vi "test code emballage_PAGO.vi"() -> ()   [LabVIEW 2011]
uses:
  <vilib>/Instr/_visa.llb/VISA Configure Serial Port (Instr).vi
panel:
  in  "Param RS232 2":T1={"VISA resource name"="COM4", "baud rate"=9600, "data bits"=8, "parity"=0, "stop bits"=10, "flow control"=0, "delay before read (ms)"=500} {"data bits" min=5 max=8 step=1; "parity" items=["Aucune", "Impaire", "Paire", "Marque", "Espace"]; "stop bits" items=["1.0"=10, "1.5"=15, "2.0"=20]; "flow control" items=["Aucune"=0, "XON/XOFF"=1, "RTS/CTS"=2, "DTR/DSR"=4]}
  in  "chaine ecrite":string
  out "chaine lue":string
  in  "Param RS232":T1={"VISA resource name"="COM4", "baud rate"=9600, "data bits"=8, "parity"=0, "stop bits"=10, "flow control"=0, "delay before read (ms)"=500} {"data bits" min=5 max=8 step=1; "parity" items=["Aucune", "Impaire", "Paire", "Marque", "Espace"]; "stop bits" items=["1.0"=10, "1.5"=15, "2.0"=20]; "flow control" items=["Aucune"=0, "XON/XOFF"=1, "RTS/CTS"=2, "DTR/DSR"=4]}
  # "ENTETE LOGO FAS MEDIC"
  # "ZB\nUS\nq592\nD7\nN\nR166,48\nI8,12,001\nGW275,824,30,55,ÿÿÿÿÿÿÿÿÿÿÿÿÿÿÿÿÿÿÿÿÿÿÿÿÿÿÿÿùÿÿÿÿÿÿÿÿÿÿÿÿÿÿÿÿÿÿÿÿÿÿÿÿÿÿÿÿÿàÿÿÿÿÿÿÿÿÿÿÿÿÿÿÿÿÿÿÿÿÿÿÿÿÿÿÿÿÿÿÿÿÿÿÿÿÿÿÿÿÿÿÿÿÿÿÿÿÿÿÿÿÿÿÿÿÿþÿÿÿÿÿÿÿÿÿÿÿÿÿÿÿÿÿÿÿÿÿÿÿÿÿÿÿø?ÿÿÿÿÿÿÿÿÿÿÿÿÿÿÿÿÿÿÿÿÿÿÿÿÿÿÿð?ÿÿÿÿÿÿÿÿÿÿÿÿÿÿÿÿÿÿÿÿÿÿÿÿÿÿÿð?ÿÿÿÿÿÿÿÿÿÿÿÿÿÿÿÿÿÿÿÿÿÿÿÿÿÿÿðÿÿÿÿÿÿÿÿÿÿÿÿÿÿÿÿÿÿÿÿÿÿÿÿÿÿÿàÿÿÿÿÿÿÿÿÿÿÿÿÿÿÿÿÿÿÿÿÿÿÿÿÿÿÿÀÿÿÿÿÿÿÿÿÿÿÿÿÿÿÿÿÿÿÿÿÿÿÿÿÿÿÿÀ?ÿàÿÿþÿàÿÿÿÿÿÿÀÿÿðÿÿÿÿÿÿÿÀ?ÿ?Ïxÿ?þóþþÀÿ?ü?þÏaàþþóø>?øüÇÏGü|Çþóð??ðüÿãÏOþxÿãþóð??àùÿóÏþ9ÿóþóàÀ??ÀÿñÿóÏÿ9ÿóþóàà???ÿóÿùÏ?ÿ3ÿùþóàà??ÿóÿùÏ?ÿÿùþóàÿþÿ?>ÿÿÿùÏÿÿùþóà?þÿ??ÿÿÿùÏÿÿùþóðþ??ÿÿÿùÏÿþóð~?ÀÿÿÿùÏÿþóøÿ?ÀÿÿÿùÏÿÿùþóþÿ?à0ÿÿÿùÏ?ÿÿùþóÿüÿÿ?ð0ÿÿÿùÏ?ÿ;ÿùüóÿÿÿÿÿ?øpÿñÿñÏÿ9ÿóüãðàÿ?ÿÿÿÿÿÿÿùÿóÏÿ9ÿóüãðÀ~`ÿÿÿÿÿÿÿùÿãÏþxÿãÏøãð`ÿÀÿüÿÇÏGü|ÇÇø?ÃðàþÀ?ÿü?ÏcðþÃãø?àþ?ÿþÏpÿð3üààüÿÿàÿÿ~ÿàÿü?áÿÿÿü?ÿ?üÿÿÿÿÿÿÿÿÿÿÿÿÿÿÿÿÿÿÿÿÿ?üÿÿÿÿÿÿÿÿÿÿÿÿÿÿÿÿÿÿÿÿÿÿ?øÿÿÿÿÿÿÿÿÿÿÿÿÿÿÿÿÿÿÿÿÿÿøÿÿÿÿÿÏÿÿÿÿÿÿÿÿÿÿÿÿÿÿÿüðÿÿÿÿÿÏÿÿÿÿÿÿÿÿÿÿÿÿÿÿÿÀðÿÿÿÿÿÏÿÿÿÿÿÿÿÿÿÿÿÿÿÿÿÀðÿÿÿÿÿÏÿÿÿÿÿÿÿÿÿÿÿÿÿÿÿÀÿàÿÿÿÿÿÏÿÿÿÿÿÿÿÿÿÿÿÿÿÿÿÀÿÀÿÿÿÿÿÿÿÿÿÿÿÿÿÿÿÿÿÿÿÿÿÿÀÿÀÿÿÿÿÿÿÿÿÿÿÿÿÿÿÿÿÿÿÿÿÿÿÿÿÿÀ0ÿÿÿÿÿÿÿÿÿÿÿÿÿÿÿÿÿÿÿÿÿÿÿÿÿ?ÿÿÿÿÿÿÿÿÿÿÿÿÿÿÿÿÿÿÿÿÿÿÿÿÿÿÿÿÿÿÿÿÿÿÿÿÿÿÿÿÿÿÿÿÿÿÿÿÿÿÿÿÿÿÿÿÿÿÿÿÿÿÿÿÿÿÿÿÿÿÿÿÿÿÿÿÿÿÿÿÿÿÿÿÿÿÿÿÿÿÿÿÿÿÿÿÿÿÿÿÿÿÿÿÿÿÿÿÿÿÿÿÿÿÿÿÿÿÿÿÿÿÿÿÿÿÿÿÿÿÿÿÿÿÿÿÿÿÿÿÿÿÿÿÿÿÿÿÿÿÿÿÿÿÿÿÿÿÿÿÿÿÿÿÀÿÿÿÿÿÿÿÿÿÿÿÿÿÿÿÿÿÿÿÿÿÿÿÿÿÿÿÿàÿÿÿÿÿÿÿÿÿÿÿÿÿÿÿÿÿÿÿÿÿÿÿÿÿÿÿÿàÿÿÿÿÿÿÿÿÿÿÿÿÿÿÿÿÿÿÿÿÿÿÿÿÿÿÿÿð?ÿÿÿÿÿÿÿÿÿÿÿÿÿÿÿÿÿÿÿÿÿÿÿÿÿÿÿÿðÿÿÿÿÿÿ\nGW62,732,54,78,ÿÿÿÿÿÿÿÿÿÿÿÿÿÿÿÿÿÿÿÿÿÿÿñÿÿüÿÿÿÿÿÿÿÿÿÿÿÿÿÿÿÿÿÿÿÿÁÿÿÿÿÿÿÿÿÿÿÿÿÿÿÿÿÿÿÿÿÿÿÿÿÿÿÿÿÿáÿÿüÿÿÿÿÿÿÿÿÿÿÿÿÿÿÿÿÿÿÿÿÿÿÿÿÿÿÿÿÿÿÿÿÿÿÿÿÿÿÿÿÿÿÿÿÿÿÿÿÿÏÿÿüÿÿÿÿÿÿÿÿÿÿÿÿÿÿÿÿÿÿÿÿÿÿÿÿÿÿÿÿÿÿÿÿÿÿÿÿÿÿÿÿÿÿÿÿÿÿÿÿÿÏ9äÌÏðçÈç<|?äó#ÏÎpùóÇ~|ÿÿÿÿÿÿÿÿÿÿÿÿÿÿÿÿÿÿÿÿÿÿÿÿ9ÀÌÎàgÈg88àsÏÎ`yó~|ÿÿÿÿÿÿÿÿÿÿÿÿÿÿÿÿÿÿÿÿÿÿÿÿ9ÌÌFgæf#Îg1Ïã3ÏÎfyó9ÿÿÿÿÿÿÿÿÿÿÿÿÿÿÿÿÿÿÿÿÿÿÿÿ9ÌÌççãæsÎg3çç39ÏÎ~yó9ÿÿÿÿÿÿÿÿÿÿÿÿÿÿÿÿÿÿÿÿÿÿÿÿ39ÌÌççðæsÎg3çç39ÏÎ`yó9ÿÿÿÿÿÿÿÿÿÿÿÿÿÿÿÿÿÿÿÿÿÿÿÿ39ÌÌççüfsÎg3çç39Î`yó99ÿÿÿÿÿÿÿÿÿÿÿÿÿÿÿÿÿÿÿÿÿÿÿÿ31ÌÌFgæf#Îf1çç39ÌfyóÿÿÿÿÿÿÿÿÿÿÿÿÿÿÿÿÿÿÿÿÿÿÿþyÀÀàg 8?çàs9ÏÀ`AÿÿÿÿÿÿÿÿÿÿÿÿÿÿÿÿÿÿÿÿÿÿÿþyÃäæOðç1<{çäó9ÏâpÁÇÿÿÿÿÿÿÿÿÿÿÿÿÿÿÿÿÿÿÿÿÿÿÿÿÿÿÿÿÿÿÿÿÿçÿþÿñÏçÿÿÏÿÿÿÿÿÿÇÿÿÿÿÿÿÿÿÿÿÿÿÿÿÿÿÿÿÿÿÿÿÿÿÿÿÿÿÿÿÿÿÿçÿþÿøçóÿÿÿÿÿÿÿÇÿÿÿÿÿÿÿÿÿÿÿÿÿÿÿÿÿÿÿÿÿÿÿÿÿÿÿÿÿÿÿÿÿçÿþÿÿü?çóÿÿÿÿÿÿÿÇÿÿÿÿÿÿÿÿÿÿÿÿÿÿÿÿÿÿÿÿÿÿÿÿÿÿÿÿÿÿÿÿÿÿÿÿÿÿÿÿÿÿÿÿÿÿÿÿÿÿÿÿÿÿÿÿÿÿÿÿÿÿÿÿÿÿÿÿÿÿÿÿÿÿÿÿÿÿÿÿÿÿÿÿÿÿÿÿÿÿÿÿÿÿÿÿÿÿÿÿÿÿÿÿÿÿÿÿÿÿÿÿÿÿÿÿÿÿÿÿÿÿÿÿÿÿÿÿÿÿÿÿÿÿÿÿÿÿÿÿÿÿÿÿÿÿÿÿÿÿÿÿÿÿÿÿÿÿÿÿÿÿÿÿÿÿÿÿÿÿÿÿÿÿÿÿÿÿÿÿÿÿÿÿÿÿÿÿÿÿÿÿÿÿÿÿÿÿÿÿÿÿÿÿÿÿÿÿÿÿÿÿÿÿÿÿÿÿÿÿÿÿÿÿÿÿÿÿÿÿÿÿÿÿÿÿÿÿÿ¿ÿÿÿÿÿÿÿÿÿÿÿÿÿÿÿÿÿÿÿýþÿÿÿÿÿÿÿÿÿÿÿÿÿÿÿÿÿÿÿïÿÿÿÿÿÿÿÿÿÿþÿßÿÿÿÿÿÿÿÿ¿ÿÿÿÿÿÿÿÿÿÿûÿÿÿÿÿÿÿÿÿÿÿÿÿÿÿÿÿÿÿßÿÿÿÿÿÿÿÿÿÿþÿßÿÿÿÿÿÿÿÿÿÿÿÿÿÿÿÿÿÿûÿÿÿÿÿÿÿÿÿÿ½Ç¸hîî÷{¿Þþ?ïïþ>>ïþñßû÷ÿÿ_Qÿxøÿ¿¿øøø¾ûÇïßÿýûÏïÿÿ½»÷§oî÷{¿þýßïïýÝÝïïþýîïû÷ÿÿîÎÿ÷w¿¿÷ww¿¿û÷»¿ïßÿÿû·ïÿÿ½½÷¯oÕjµ_þûïïïûëëïïýýßoû÷ýÿõÞÿï¯¿¿¿ï¯¯¿¿÷÷}¿ïß÷ÿû{ïÿÿ½ý÷ïoÕjµ_þûïïïûëëÿïûýßoûà}ÿõÞÿï¯¿¿¿ï¯¯ÿ¿ï÷}¿ï÷ÿûûïÿÿ½ýùèïÕjµ_þûïïïûëê?ï÷ýßoû÷}ÿûÑÿï¯¿¿¿ï¯¨ÿ¿ß÷}¿ïÝ÷ÿûïÿÿ½ýþgïÕjµ_þûïïïýÛéßïïýßoûöà?õÏÿï¯¿¿¿÷o§¿¿÷}¿ïÛÿû{ïÿÿ½½÷¯oÕjµ_þûïïïþ;ëïïßýßoûöýÿõÞàï¯¿¿¿øï¯¿¿÷}¿ïÛ÷ÿû{ïÿÿ¹»÷·o»Îïþ»ïëëýÛëïë¿ýßoúõýÿîîÿï¯¿¯¯÷o¯¿®ÿ÷}¿ë×÷ÿû·ïÿÿÅÇøxÇ»Îïþ{ïççûëëïç¾þß_ùõýÿ_qÿï¯¿ï¯¯¿ûû}ç×÷ýûÏïÿÿýÿÿÿïÿÿÿÿþ{ïççûëëïç¾þß_ùóÿÿÿÿÿï¯¿ï¯¯¿ûû}çÏÿÿûÿïÿÿýÿÿÿïÿÿÿÿþýßïïýÝÝßïÝþîßû÷ÿÿÿÿÿ÷w¿¿÷ww¿wû»ïßÿÿûÿïÿÿýÿÿÿÿÿÿÿþþ?ïïþ>>?ïãÿq¿û÷ÿÿÿÿÀøøÿ¿¿øøøÿ¿ýÆÿïßÿÿûÿÿÿÿÿÿÿÿÿÿÿÿÿÿÿÿÿÿÿÿÿÿÿÿÿÿÿÿÿÿÿÿÿÿÿÿÿÿÿÿÿÿÿÿÿÿÿÿÿÿÿÿÿÿÿÿÿÿÿÿÿÿÿÿÿÿÿÿÿÿÿÿÿÿÿÿÿÿÿÿÿÿÿÿÿÿÿÿÿÿÿÿÿÿÿÿÿÿÿÿÿÿÿÿÿÿÿÿÿÿÿÿÿÿÿÿÿÿÿÿÿÿÿÿÿÿÿÿÿÿÿÿÿÿÿÿÿÿÿÿÿÿÿÿÿÿÿÿÿÿÿÿÿÿÿÿÿÿÿÿÿÿÿÿÿÿÿÿÿÿÿÿÿÿÿÿÿÿÿÿÿÿÿÿÿÿÿÿÿÿÿÿÿÿÿÿÿÿÿÿÿÿÿÿÿÿÿÿÿÿÿÿÿÿÿÿÿÿÿÿÿÿÿÿÿÿÿÿÿÿÿÿÿÿÿÿÿÿÿÿÿÿÿÿÿÿÿÿÿÿÿÿÿÿÿÿÿÿÿÿÿÿÿÿÿÿÿÿÿÿÿÿÿÿÿÿÿÿÿÿÿÿÿÿÿÿÿÿÿÿÿÿÿÿÿÿÿÿÿÿÿÿÿÿÿÿÿÿÿÿÿÿÿÿÿÿÿÿÿÿÿÿÿÿÿÿÿÿÿÿÿÿÿÿÿÿÿÿÿÿÿÿÿÿÿÿÿÿÿÿÿÿÿÿÿÿÿÿÿÿÿÿÿÿÿÿÿÿÿÿÿÿÿÿÿÿÿÿÿÿÿÿÿÿÿÿÿÿÿÿÿÿÿÿÿÿÿÿÿÿÿÿÿÿÿÿÿÿÿÿÿÿÿÿÿÿÿÿÿÿÿÿÿÿÿÿÿÿÿÿÿÿÿÿÿÿÿÿÿÿÿÿÿÿÿÿÿÿÿÿÿÿÿÿÿÿÿÿÿÿÿÿÿÿÿÿÿÿÿÿÿÿþÿÿÿÿÿÿÿÿÿÿÿÿÿÿÿÿÿÿÿÿÿÿÿÿÿÿÿÿÿÿÿÿþÿÿÿÿÿÿÿÿÿÿÿÿÿÿÿÿÿÿÿÿýÿÿÿÿÿÿÿÿÿÿÿÿÿÿÿÿÿÿÿÿÿÿÿéïhïyà»ãþóöýõ=Ïhÿ¿ûÇÇßû÷ýç·ôá£§½¿Ï{Ïÿÿÿÿÿÿÿÿÿÿæïgovÿ[»ÝÿíövûþìîÝý·g¿û»»ßû÷wÿÛ·nöÞ½¿·{·þÿÿÿÿÿÿÿÿÿÿïoooo~ÛU¾ÿÞööýÿ]ííû{o¿û}}ßûöûÿ½¶ööÞ½½½¿{{{ýÿÿÿÿÿÿÿÿÿÿïooo}ÛU¾ÿþööþÿ]ïí÷ûo¿÷}}ßûöýÿý·ööß½½½¿û{{ûÿÿÿÿÿÿÿÿÿÿïohï`}ÛU¿ÿÀöþÃ½ì\n÷hÿ¿÷}}ß÷ýÿ¶öç½½½¿{{ûÿÿÿÿÿÿÿÿÿÿïogïo{ÛUÏÿÞö~ÿ]ííï{gð?÷}}ßû÷ýÿ½¶ööù½½½¿{{{÷ÿÿÿÿÿÿÿÿÿÿïoooowÛUñÿÞö÷þÿ]ííß{oo¿ï}¹ßøýÿ½¶ööÞ½½½¿{{{ïÿÿÿÿÿÿÿÿÿÿæîwjvïÚîþÿí§wþþíîÝ¿·wo¿ï}Å×û÷ýÿÛ·n¦Þ½¹¿·s·Ïÿÿÿÿÿÿÿÿÿÿéñxéyà\nî¾ÿóþýõï=Ïxï¿ß}ýÏûöýÿç·a½§Å¿ÏÏßÿÿÿÿÿÿÿÿÿÿïÿÿïÿÿßÿ¾ÿÿÿþýÿÿÿÿÿÿï¿¿}}Ïûöûÿÿ·ÿþÿÿ¿ÿ¿ÿÿÿ¿ÿÿÿÿÿÿÿÿÿÿïÿÿïÿÿßÿÝÿÿÿÿ{ÿÿÿÿÿÿï¿»{ßû÷wÿÿ·ÿþÿÿ¿ÿ¿ÿÿÿÿÿÿÿÿÿÿÿÿÿïÿÿïÿÿÛÿãÿÿÿÿÿÿÿýÿÿð?Çßû÷ÿÿ·þþÿÿ¿ÿ¿ÿÿÿÿÿÿÿÿÿÿÿÿÿÿÿÿÿÿÿÿÿÿÿÿÿÿÿÿÿÿÿÿÿÿÿÿÿÿÿÿÿÿÿÿÿÿÿÿÿÿÿÿÿÿÿÿÿÿÿÿÿÿÿÿÿÿÿÿÿÿÿÿÿÿÿÿÿÿÿÿÿÿÿÿÿÿÿÿÿÿÿÿÿÿÿÿÿÿÿÿÿÿÿÿÿÿÿÿÿÿÿÿÿÿÿÿÿÿÿÿÿÿÿÿÿÿÿÿÿÿÿÿÿÿÿÿÿÿÿÿÿÿÿÿÿÿÿÿÿÿÿÿÿÿÿÿÿÿÿÿÿÿÿÿÿÿÿÿÿÿÿÿÿÿÿÿÿÿÿÿÿÿÿÿÿÿÿÿÿÿÿÿÿÿÿÿÿÿÿÿÿÿÿÿÿÿÿÿÿÿÿÿÿÿÿÿÿÿÿÿÿÿÿÿÿÿÿÿÿÿÿÿÿÿÿÿÿÿÿÿÿÿÿÿÿÿÿÿÿÿÿÿÿÿÿÿÿÿÿÿÿÿÿÿÿÿÿÿÿÿÿÿÿÿÿÿÿÿÿÿÿÿÿÿÿÿÿÿÿÿÿÿÿÿÿÿÿÿÿÿÿÿÿÿÿÿÿÿÿÿÿÿÿÿÿÿÿÿÿÿÿÿÿÿÿÿÿÿÿÿÿÿÿÿÿÿÿÿÿÿÿÿÿÿÿÿÿÿÿÿÿÿÿÿÿÿÿÿÿÿÿÿÿÿÿÿÿÿÿÿÿÿÿÿÿÿÿÿÿÿÿÿÿÿÿÿÿÿÿÿÿÿÿÿÿÿÿÿÿÿÿÿÿÿÿÿÿÿÿÿÿÿÿÿÿÿÿÿÿÿÿÿÿÿÿÿÿÿÿÿÿÿÿÿÿÿÿÿÿÿÿÿÿÿÿÿÿÿÿÿÿÿÿÿÿÿÿÿÿÿÿÿÿÿÿÿÿÿÿÿÿÿÿÿÿÿÿÿÿÿÿÿÿÿÿÿÿÿÿÿÿÿÿÿÿÿÿÿÿÿÿÿÿÿÿÿÿÿÿÿÿÿÿÿÿÿÿÿÿÿÿÿÿÿÿÿÿÿÿÿÿÿÿÿÿÿÿÿÿÿÿÿÿÿÿÿÿÿÿÿÿÿÿÿÿÿÿÿÿÿÿÿÿÿÿÿÿÿÿÿÿÿÿÿÿÿÿÿÿÿÿÿÿÿýoñÚ~{Þÿýýÿÿÿÿÿÿÿÿÿÿÿÿÿÿÿÿÿÿÿÿÿÿÿÿÿÿÿÿÿÿÿÿÿÿÿÿÿÿÿÿÿÿ~ïîÙ½»®þíýýÿÿÿÿÿÿÿÿÿÿÿÿÿÿÿÿÿÿÿÿÿÿÿÿÿÿÿÿÿÿÿÿÿÿÿÿÿÿÿÿÿÿ¾ý÷ï[ÛÛ®ýöûýÿÿÿÿÿÿÿÿÿÿÿÿÿÿÿÿÿÿÿÿÿÿÿÿÿÿÿÿÿÿÿÿÿÿÿÿÿÿÿÿÿÿ¾ý÷ÿ[ßÛ®ýöûýÿÿÿÿÿÿÿÿÿÿÿÿÿÿÿÿÿÿÿÿÿÿÿÿÿÿÿÿÿÿÿÿÿÿÿÿÿÿÿÿÿÿýÿÿ[ØvýþýÿÿÿÿÿÿÿÿÿÿÿÿÿÿÿÿÿÿÿÿÿÿÿÿÿÿÿÿÿÿÿÿÿÿÿÿÿÿÿÿÿÿÝþÿ[ÛÛvþwýÿÿÿÿÿÿÿÿÿÿÿÿÿÿÿÿÿÿÿÿÿÿÿÿÿÿÿÿÿÿÿÿÿÿÿÿÿÿÿÿÿÿÝÿï[ÛÛvÿwÿÿÿÿÿÿÿÿÿÿÿÿÿÿÿÿÿÿÿÿÿÿÿÿÿÿÿÿÿÿÿÿÿÿÿÿÿÿÿÿÿÿÝÿ÷îÙ½ºúÿ÷wýÿÿÿÿÿÿÿÿÿÿÿÿÿÿÿÿÿÿÿÿÿÿÿÿÿÿÿÿÿÿÿÿÿÿÿÿÿÿÿÿÿÿëý÷ñÚ~zúý÷¯ýÿÿÿÿÿÿÿÿÿÿÿÿÿÿÿÿÿÿÿÿÿÿÿÿÿÿÿÿÿÿÿÿÿÿÿÿÿÿÿÿÿÿëý÷ÿûÿúúý÷¯ýÿÿÿÿÿÿÿÿÿÿÿÿÿÿÿÿÿÿÿÿÿÿÿÿÿÿÿÿÿÿÿÿÿÿÿÿÿÿÿÿÿÿëþïÿûÿùüþï¯ýÿÿÿÿÿÿÿÿÿÿÿÿÿÿÿÿÿÿÿÿÿÿÿÿÿÿÿÿÿÿÿÿÿÿÿÿÿÿÿÿÿÿ÷ÿÿÛÿùüÿßÿ\nP1"
  # "Grande etiquette - 1 code bar 2D + scan"
  # "Grande etiquette - 1 code bar 2D"
  # "ZB\nUS\nq592\nD7\nN\nR166,48\nI8,12,001\nA500,828,2,1,1,1,N,\"FASmedic s.a.\"\nA500,812,2,1,1,1,N,\"Zone industrielle\"\nA500,796,2,1,1,1,N,\"CH-1607 Pal‚zieux-Gare\"\nA500,780,2,1,1,1,N,\"T‚l.+41(0)21 907 79 71\"\nA500,764,2,1,1,1,N,\"www.fasmedic.com\"\nA10,712,3,2,1,1,N,\"Destinataire:Respironics\"\nA34,712,3,2,1,1,N,\"Nшcommande:XXXXXXXX\"\nA58,712,3,2,1,1,N,\"Carton:1/2\"\nA82,712,3,2,1,1,N,\"Quantit‚:50/100\"\nA106,712,3,2,1,1,N,\"Votre ref.:ZZZZZ\"\nA162,712,3,2,1,1,N,\"Nшvalves:\"\nA162,592,3,1,1,1,N,\"08120001, 08120002, 08120003, 08120004, 08120005\"\nA178,592,3,1,1,1,N,\"08120006, 08120007, 08120008, 08120009, 08120010\"\nA194,592,3,1,1,1,N,\"08120011, 08120012, 08120013, 08120014, 08120015\"\nA210,592,3,1,1,1,N,\"08120016, 08120017, 08120018, 08120019, 08120020\"\nA226,592,3,1,1,1,N,\"08120021, 08120022, 08120023, 08120024, 08120025\"\nA242,592,3,1,1,1,N,\"08120026, 08120027, 08120028, 08120029, 08120030\"\nA258,592,3,1,1,1,N,\"08120031, 08120032, 08120033, 08120034, 08120035\"\nA274,592,3,1,1,1,N,\"08120036, 08120037, 08120038, 08120039, 08120040\"\nA290,592,3,1,1,1,N,\"08120041, 08120042, 08120043, 08120044, 08120045\"\nA306,592,3,1,1,1,N,\"08120046, 08120047, 08120048, 08120049, 08120050\"\nA186,696,3,2,1,1,N,\"(P/N)\"\nLO358,112,2,600\nb392,608,D,4,\"12-216C-04521 F120078 417mA 14.4ohm     03838/08-07.01.01\"\nA392,592,3,2,1,1,N,\"Nшarticle FAS:\"\nA420,592,3,3,1,1,N,\"12-216C-04521 F120078 417mA 14.4ohm\"\nA448,592,3,2,1,1,N,\"Nшcommande FAS:\"\nA476,592,3,3,1,1,N,\"03838/08-07.01.01\"\nB358,64,2,1,1,2,56,N,\"ZZZZZ 03 08010801 50\"\nA358,0,2,3,1,1,N,\"ZZZZZ 08010801 50\"\nGW265,824,32,61,яяяяяяяяяяяяяяяяяяяяяяяяяяяяяяяЏяяяяяяяяяяяяяяяяяяяяяяяяяяяяяяюяяяяяяяяяяяяяяяяяяяяяяяяяяяяяяшяяяяяяяяяяяяяяяяяяяяяяяяяяяяяяАяяяяяяяяяяяяяяяяяяяяяяяяяяяяяяяяяяяяяяяяяяяяяяяяяяяяяяяяяяяяяяяяяяяяяяяяяяяяяяяяяяяяяяяяяюяяяяяяяяяяяяяяяяяяяяяяяяяяяяяюяяяяяяяяяяяяяяяяяяяяяяяяяяяяяюяяяяяяяяяяяяяяяяяяяяяяяяяяяяяьяяяяяяяяяяяяяяяяяяяяяяяяяяяяяьяяяяяяяяяяяяяяяяяяяяяяяяяяяяяшяЃяяяяьяяяяяяаяяяЂ?яяяяяяяшюП<ярьящяуя?Аяю8ш>П0x?БрьящяуьАяь0щяЏП#яЏь|ящяушАяшpуяЗП'яЏю<ящяурАяр`гягПяЏ?яящяуарАшяаазяуПяЗ?яњящяуашАьяЂАЗяуПяж?яњящяуашАьяАПяыПяжяЬящяуаяяАья~АяящПязяяМящяуаяяАшяЂяящП?язяяМящяуаяАаяЂяящП?ячяяМящяур?АяЂ?яящП?яцящяурАяА?яящП?яцящяушАяаяящП?яжяМящяуяАяряящПяжяЬящяуярАяяряяыПяжяњящягяяаАяяяшяПяуПяж?яњящягррАяяяяяяяяяяЗяуПяЗ?яясягррАшяяяяяяязягПяП?я>ясягрраряЂягязП'яЏџю>аяГраяЂ0ясяЏП#я‡ь~?А“шря0яшяП1ь?ГряЊ3ьшюpяь?П8аяЂsьью`яяЃяя?ѓяюяаяГяяАяяАяяьаяяяяя?яяяяяяяяяяяяяяяяяяьАяяяяя?яяяяяяяяяяяяяяяяяюьАяяяяя?яяяяяяяяяяяяяяяяяюшАяяяяя?яяяяяяяяяяяяяяяяяьшЂяяяяП?яяяяяяяяяяяяяяяяярЂяяяяП?яяяяяяяяяяяяяяяяяяр?яяяяП?яяяяяяяяяяяяяяяяяяр?яяяяП?яяяяяяяяяяяяяяяяяяаяяяяП?яяяяяяяяяяяяяяяяяяаяяяяяяяяяяяяяяяяяяяяяяяяАяяяяяяяяяяяяяяяяяяяяяяяяяяяАяяяяяяяяяяяяяяяяяяяяяяяяяяяЂяяяяяяяяяяяяяяяяяяяяяяяяяяяяяЂяяяяяяяяяяяяяяяяяяяяяяяяяяяяяЂ?яяяяяяяяяяяяяяяяяяяяяяяяяяяяяЂ?яяяяяяяяяяяяяяяяяяяяяяяяяяяяяЂ?яяяяяяяяяяяяяяяяяяяяяяяяяяяяяЂяяяяяяяяяяяяяяяяяяяяяяяяяяяяяАяяяяяяяяяяяяяяяяяяяяяяяяяяяяяаяяяяяяяяяяяяяяяяяяяяяяяяяяяяяяаяяяяяяяяяяяяяяяяяяяяяяяяяяяяяяряяяяяяяяяяяяяяяяяяяяяяяяяяяяяяр?яяяяяяяяяяяяяяяяяяяяяяяяяяяяяяшяяяяяяяяяяяяяяяяяяяяяяяяяяяяяящяяяяяя\nP1"
  # "ZB\nUS\nq592\nD7\nN\nR166,48\nI8,12,001\nA504,828,2,1,1,1,N,\"FASmedic s.a.\"\nA504,812,2,1,1,1,N,\"Zone industrielle\"\nA504,796,2,1,1,1,N,\"CH-1607 Pal‚zieux-Gare\"\nA504,780,2,1,1,1,N,\"T‚l.+41(0)21 907 79 71\"\nA504,764,2,1,1,1,N,\"www.fasmedic.com\"\nA34,712,3,2,1,1,N,\"Destinataire:EMS Electro Medical System\"\nA74,712,3,2,1,1,N,\"Nшcommande:CF-08-0253/2\"\nA114,712,3,2,1,1,N,\"Carton:1/2\"\nA154,712,3,2,1,1,N,\"Quantit‚:50/100\"\nA194,712,3,2,1,1,N,\"Votre ref.:EL-360\"\nLO258,112,2,600\nb404,112,D,4,\"12-216C-04521 EQIFIL 417mA 14.4ohm     03838/08-07.01.01\"\nA318,712,3,2,1,1,N,\"Nшarticle FAS:\"\nA358,712,3,3,1,1,N,\"12-216C-04521 EQIFIL 417mA 14.4ohm\"\nA398,712,3,2,1,1,N,\"Nшcommande FAS:\"\nA438,712,3,3,1,1,N,\"03838/08-07.01.01\"\nB318,64,2,3,1,2,56,N,\"EL-360 03 08010801\"\nA318,0,2,3,1,1,N,\"EL-360 03 08010801\"\nGW265,824,32,61,яяяяяяяяяяяяяяяяяяяяяяяяяяяяяяяЏяяяяяяяяяяяяяяяяяяяяяяяяяяяяяяюяяяяяяяяяяяяяяяяяяяяяяяяяяяяяяшяяяяяяяяяяяяяяяяяяяяяяяяяяяяяяАяяяяяяяяяяяяяяяяяяяяяяяяяяяяяяяяяяяяяяяяяяяяяяяяяяяяяяяяяяяяяяяяяяяяяяяяяяяяяяяяяяяяяяяяяюяяяяяяяяяяяяяяяяяяяяяяяяяяяяяюяяяяяяяяяяяяяяяяяяяяяяяяяяяяяюяяяяяяяяяяяяяяяяяяяяяяяяяяяяяьяяяяяяяяяяяяяяяяяяяяяяяяяяяяяьяяяяяяяяяяяяяяяяяяяяяяяяяяяяяшяЃяяяяьяяяяяяаяяяЂ?яяяяяяяшюП<ярьящяуя?Аяю8ш>П0x?БрьящяуьАяь0щяЏП#яЏь|ящяушАяшpуяЗП'яЏю<ящяурАяр`гягПяЏ?яящяуарАшяаазяуПяЗ?яњящяуашАьяЂАЗяуПяж?яњящяуашАьяАПяыПяжяЬящяуаяяАья~АяящПязяяМящяуаяяАшяЂяящП?язяяМящяуаяАаяЂяящП?ячяяМящяур?АяЂ?яящП?яцящяурАяА?яящП?яцящяушАяаяящП?яжяМящяуяАяряящПяжяЬящяуярАяяряяыПяжяњящягяяаАяяяшяПяуПяж?яњящягррАяяяяяяяяяяЗяуПяЗ?яясягррАшяяяяяяязягПяП?я>ясягрраряЂягязП'яЏџю>аяГраяЂ0ясяЏП#я‡ь~?А“шря0яшяП1ь?ГряЊ3ьшюpяь?П8аяЂsьью`яяЃяя?ѓяюяаяГяяАяяАяяьаяяяяя?яяяяяяяяяяяяяяяяяяьАяяяяя?яяяяяяяяяяяяяяяяяюьАяяяяя?яяяяяяяяяяяяяяяяяюшАяяяяя?яяяяяяяяяяяяяяяяяьшЂяяяяП?яяяяяяяяяяяяяяяяярЂяяяяП?яяяяяяяяяяяяяяяяяяр?яяяяП?яяяяяяяяяяяяяяяяяяр?яяяяП?яяяяяяяяяяяяяяяяяяаяяяяП?яяяяяяяяяяяяяяяяяяаяяяяяяяяяяяяяяяяяяяяяяяяАяяяяяяяяяяяяяяяяяяяяяяяяяяяАяяяяяяяяяяяяяяяяяяяяяяяяяяяЂяяяяяяяяяяяяяяяяяяяяяяяяяяяяяЂяяяяяяяяяяяяяяяяяяяяяяяяяяяяяЂ?яяяяяяяяяяяяяяяяяяяяяяяяяяяяяЂ?яяяяяяяяяяяяяяяяяяяяяяяяяяяяяЂ?яяяяяяяяяяяяяяяяяяяяяяяяяяяяяЂяяяяяяяяяяяяяяяяяяяяяяяяяяяяяАяяяяяяяяяяяяяяяяяяяяяяяяяяяяяаяяяяяяяяяяяяяяяяяяяяяяяяяяяяяяаяяяяяяяяяяяяяяяяяяяяяяяяяяяяяяряяяяяяяяяяяяяяяяяяяяяяяяяяяяяяр?яяяяяяяяяяяяяяяяяяяяяяяяяяяяяяшяяяяяяяяяяяяяяяяяяяяяяяяяяяяяящяяяяяя\nP1"
  # "Grande etiquette - 2 code bar 1D"
  # "LOGO fluid autom syst en noir et blanc rotation 180°"
  # "ZB\nUS\nq592\nD7\nN\nR166,48\nI8,12,001\nA82,429,3,1,1,1,N,\"FASmedic s.a.\"\nA98,429,3,1,1,1,N,\"Zone industrielle\"\nA114,429,3,1,1,1,N,\"CH-1607 Pal‚zieux-Gare\"\nA130,429,3,1,1,1,N,\"T‚l.+41(0)21 907 79 71\"\nA146,429,3,1,1,1,N,\"www.fasmedic.com\"\nA33,856,3,2,1,1,N,\"Client : Saime\"\nA78,856,3,2,1,1,N,\"Commande : 01054/08-01.01.01\"\nA126,856,3,2,1,1,N,\"Carton : 1/2\"\nA171,856,3,2,1,1,N,\"Nb de valves : 50\"\nA216,856,3,2,1,1,N,\"Nш valves :\"\nA216,712,3,1,1,1,N,\"08120001, 08120002, 08120003, 08120004, 08120005\"\nA232,712,3,1,1,1,N,\"08120006, 08120007, 08120008, 08120009, 08120010\"\nA248,712,3,1,1,1,N,\"08120011, 08120012, 08120013, 08120014, 08120015\"\nA264,712,3,1,1,1,N,\"08120016, 08120017, 08120018, 08120019, 08120020\"\nA280,712,3,1,1,1,N,\"08120021, 08120022, 08120023, 08120024, 08120025\"\nA296,712,3,1,1,1,N,\"08120026, 08120027, 08120028, 08120029, 08120030\"\nA312,712,3,1,1,1,N,\"08120031, 08120032, 08120033, 08120034, 08120035\"\nA328,712,3,1,1,1,N,\"08120036, 08120037, 08120038, 08120039, 08120040\"\nA344,712,3,1,1,1,N,\"08120041, 08120042, 08120043, 08120044, 08120045\"\nA360,712,3,1,1,1,N,\"08120046, 08120047, 08120048, 08120049, 08120050\"\nA240,840,3,2,1,1,N,\"(P/N)\"\nB406,800,3,1,1,2,56,N,\"12-216C-04521 EQIFIL 417mA 14.4ohms\"\nA470,806,3,3,1,1,N,\"12-216C-04521 EQIFIL 417mA 14.4\"\nA467,370,3,4,1,1,N,\"Х\"\nB438,128,2,3,1,2,56,N,\"MK3845ZZ45988 03 08120812 50\"\nA438,64,2,3,1,1,N,\"MK3845ZZ45988 03 08120812 50\"\nGW16,196,10,254,яяяяяЏяяяяяяяшѓяяяяяяярбяяяяяяягяшяяяяяяязяьяяяяяяпяюяяяяяяПяя?яяяяяяПяя?яяяяяяПяя?яяяяяяЯяя?яяяяяяЯяя?яяяяяяПяя?яяяяяяПяя?яяяяяяПяя?яяяяяязяю?яяяяяязяюяяяяяягяьяяяяяяряряяяяяяяш?БяяяяяяяюяяяяяяяяА?яяяяяяяяяяяяяяяяяяяяяяяяяяяяяяяяяяяяѓА?яяяяяѓА?яяяяяяяяяяяяяяяяяяяяяяяяяяяяяяяяяяяяяяяяяяяяяЂ?яяяяяЂ?яяяяяяьѓяяяяяяяшбяяяяяяяуяьяяяяяяягяьяяяяяязяюяяяяяяПяя?яяяяяяПяя?яяяяяяПяя?яяяяяяЯяя?яяяяяяПяя?яяяяяяПяя?яяяяяяПяя?яяяяяяПяя?яяяяяязяюяяяяяягяьяяяяяябяшяяяяяяшбяяяяяяяьяяяяяяяяяяяяяяяяяяяяяяяяяяяяяяяяяяяяПяяяяяяяьГяяяяяяяш{аяяяяяяясыьяяяяяягыьяяяяяязыюяяяяяяПыя?яяяяяяПыя?яяяяяяПыя?яяяяяяПыя?яяяяяяЯыя?яяяяяяПыя?яяяяяяПыя?яяяяяяПыя?яяяяяязыюяяяяяягыюяяяяяябыьяяяяяяшыряяяяяяяш;Бяяяяяяяюяяяяяяяяаяяяяяяяяяяяяяяяяяяяяяяяяяяяю?яяяяяяр?яяяяяябяяяяяяяяягяяяяяяяяяПяяяяяяяяяПяяяяяяяяяПяяяяяяяяяПяяяяяяяяяПяяяяяяяяяПяяяяяяяяяПяяяяяяяяяпяяяяяяяяязяяяяяяяяяуяяяяяяяяяшяяяяяяяяяш?яяяяяяр?яяяяяябяяяяяяяяязяяяяяяяяяПяяяяяяяяяПяяяяяяяяяПяяяяяяяяяЯяяяяяяяяяПяяяяяяяяяПяяяяяяяяяПяяяяяяяяязяяяяяяяяягяяяяяяяяясяяяяяяяяяш?яяяяяяяяА?яяяяяяА?яяяяяяяяяяяяяяяяяяяяяяяяяяяяяяяяяяяяяяяяяяяяяяяяяяяяяяяяяяяяяяяяяш|яяяяяяярxяяяяяяяаxяяяяяяаpяяяяяяаpяяяяяяАp?яяяяяяА`?яяяяяяА`?яяяяяяЂ`?яяяяяяЂа8?яяяяяяЃаxяяяяяяѓа|яяяяяяѓа|яяяяяяѓА|яяяяяяѓА|яяяяяяЃАшяяяяяяЂряяяяяяАА?яяяяяяАА?яяяяяяАА?яяяяяяАА?яяяяяяаА?яяяяяяаАяяяяяярАяяяяяяшАяяяяяяяюБяяяяяяяяяПяяяяяяяяяяяяяяяяяяяяяяяяяяяяяяяяяяяяяя?яяяяяяь?яяяяяяр?яяяяяяа?яяяяяяа?яяяяяяа?яяяяяяА?яяяяяяА?яяяяяяА?яяяяяяА`ЃяяяяяяяЂбаяяяяяяяЃбаяяяяяяѓбряяяяяяѓбш?яяяяяяѓаш?яяяяяяѓаш?яяяяяяѓаьяяяяяяЃашяяяяяяЂашяяяяяяА`pяяяяяяА`яяяяяяА`яяяяяяА`?яяяяяяа`?яяяяяяаp?яяяяяярpяяяяяяшxяяяяяяшxяяяяяяяьяяяяяяяяяяяяяяяАяяяяяяяяАяяяяяяяяАяяяяяяяяАяяяяяяяяАяяяяяяяяАяяяяяяяяАяяяяяяяяАяяяяяяяя?яяяяя?яяяяя?яяяяя?яяяяяЂ?яяяяяЂ?яяяяяА?яяяяяа?яяяяяш?яяяяяяАяяяяяяяяяАяяяяяяяяяАяяяяяяяяяАяяяяяяяяяАяяяяяяяяяАяяяяяяяяяяяїяяяяяяяяяяяяяяяяьяяяяюяяшяяяяш?яряяяяаяаяяяяАяАяяяяА?АяяяАА?яяяаА?яяяаА?яяярА?яяярА?яяяшА?яяяшА?яяяьА?яяяьА?яяяяА?яяяяЂА?яяяярА?яяяяьА?яяяяяА?яяяяяаА?яяяяьшА?яяяяьА?яяяяьБА?яяяяьсА?яяяяь}А?яяяяьА?яяяяьа?яяяяьь?яяяяьџ?яяяяьѓА?яяяяьЂш?яяяяьЂ~?яяяяьЂяяяяяьЂяяяяяьАяяяяьАяяяяьАяяяяьАяяяяА?яяяяААяяяяшАяяяяяАяяяяяБАяяяяябАяяяяяэАяяяяяяАяяяяяяаяяяяяяшяяяяяяяяяяяяяяаяяяяяяяшяяяяяяяьяяяяяяяяЂяяяяяяяябяя\nP1"
  # "GW0,824,67,55,яяяяяяяяяяяяяяяяяяяяяяяяяяяяяяяяяяяяяяяяяяяяяяяяяяяяяяяяяяяяяяяяябяяяяяяяяяяяяяяяяяяяяяяяяяяяяяяяяяяяяяяяяяяяяяяяяяяяяяяяяяяяяяяяяяяЃяяяяяяяяяяяяяяяяяАяяяяяяяяяяяяяяяяяяяяяяяяяяяяяяяяяяяяяяяяяяяяяяюяяяяяяяяяяяяяяяяяяяяяяяяяяяяяяяяяяяяяяяяяяяяяяяяяяяяяяяяяяяяяяяшяяяяяяяяяяяяяяяяюяяяяяяяяяяяяяяяяяяяяяяяяяяяяяяяяяяяяяяяяяяяяяяряяяяяяяяяяяяяяяьяяяяяяяяяяяяяяяяяяяяяяяяяяяяяяяяяяяяяяяяяяяяяяа?яяяяяяяяяяяяяяяьяяяяяяяяяяяяяяяяяяяяяяяяяяяяяяяяяяяяяяяяяяяяяяяа?яяяяяяяяяяяяяяяьяяяяяяяяяяяяяяяяяяяяяяяяяяяяяяяяяяяяяяяяяяяяяяяаяяяяяяяяяяяяяяяшяяяяяяяяяяяяяяяяяяяяяяяяяяяяяяяяяяяяяяяяяяяяяяяАяяяяяяяяяяяяяяяш?яяяяяяяяяяяяяяяяяяяяяяяяяяяяяяяяяяяяяяяяяяяяяяяА?яЂ?Аюр?А?аьяряАяьаашр<ашшьрxАр?яш8р>ьаяяяяЂ?юАюр?АрряяьаЂшш0ашашр`аАяш р>ьаьЂьАюр>Аа?рюяьашшашАxраяшр>|ашшАюр<ААаьяьа~шшашЂ8раяшр>|арярАюр8ЂЬЂшашЂяьа|ЂшАшЂаша;ЃраяшЂр>а<ааяр?ЏАюр?АьЃьбшЗяьаxАxАшАашрЃра?яшАр>а<аАяр?яАюр?яАьЃяяБшяяьаxаxАшАашшЃр?ЃаяшАр>р<аЂяряАюр?яа|ЂяяБшяяьаp?р8АшАашьЃр?Ѓаяшаp>р<аяряАюр?яа|Ђяѓѓшяяьаp?р8АшЃашьЃр?Ѓа~яшаp>р<а~яш?Аюр8|Аяѓѓьяьаp?р8АшашьЃр?Ѓа`яшаp>р<аяьАюр8|аѓѓюяьаp?р8АшашьЃр?Ѓаяшаp>р<аяяЂАюр8|ь?ЃяАяьаp?р8Аш?ашьЃр?Ѓаяяшаp>р<аЂяярАюр8а|яЂБяшяьаp?р8АшяашьЃр?Ѓаяяшаp>р<аЂ0яяюАюр8а|ярБяяяьаp?р8АшяашьЃр?Ѓаяяшаp>р<аА0яяяАьр<АьяшАяяЃяьаxаxАшза~шшЃр?ЃаџяшАp>р<аа яяАьа<АьшшаяЏЃяьАxАxАшБа~ррЃр?ЃаяшАр>р<ар`яшАxА>ЂьАpа|яьЂ|ЂшАшѓа<аа?Ѓр?Ѓа>яшЂр>р<аяяяяяяяьа>Аа<а~яю~шрЂ80?Ѓряшр>р<яяяяяяяьа?Аа<р~яюшрЂАш0?Ѓряшр>р<юА?яюрЂ?ЂАрxр?яя0ЂшшАаш0?Ѓш?яшр>р<юЂ?яяЂ?ьаx?рАьшр?АяяАрашЂ?юр<шш0?Ѓюяяшр>р<ьЂяяяяяяяяяяяьяяяяяяяяяяяяяяяяяАяяяяяяяяяяяЃяяяяяяяшяяяяяьаьяяяяяяяяяяяьяяяяяяяяяяяяяяяяяАяяяяяяяяяяяЃяяяяяяяшяяяяяьаьяяяяяяяяяяяяьяяяяяяяяяяяяяяяяяАяяяяяяяяяяяЃяяяяяяяшяяяяяьашяяяяяяяяяяяяьяяяяяяяяяяяяяяяяяАяяяяяяяяяяяЃяяяяяяяшяяяяяьАшяяяяяяяяяяяяьяяяяяяяяяяяяяяяшБяяяяяяяяяяяѓяяяяяяяшяр?яяьряяяяяяяяяяяяьяяяяяяяяяяяяяяяшЗяяяяяяяяяяяЏяяяяяяяшяр?яяьяряяяяяяяяяяяяэяяяяяяяяяяяяяяяяшЯяяяяяяяяяяяїяяяяяяяшяр?яяьяаяяяяяяяяяяяяяяяяяяяяяяяяяяяяяшяяяяяяяяяяяяяяяяяяяяшяр?яяьяаяяяяяяяяяяяяяяяяяяяяяяяяяяяяяяяяяяяяяяяяяяяяяяяяяяяяяяяяяяяяяяаяяяяяяяяяяяяяяяяяяяяяяяяяяяяяяяяяяяяяяяяяяяяяяяяяяяяяяяяяяяяяяАяяяяяяяяяяяяяяяяяяяяяяяяяяяяяяяяяяяяяяяяяяяяяяяяяяяяяяяяяяяяяяА0яяяяяяяяяяяяяяяяяяяяяяяяяяяяяяяяяяяяяяяяяяяяяяяяяяяяяяяяяяяяяяЂ0яяяяяяяяяяяяяяяяяяяяяяяяяяяяяяяяяяяяяяяяяяяяяяяяяяяяяяяяяяяяяяЂ0яяяяяяяяяяяяяяяяяяяяяяяяяяяяяяяяяяяяяяяяяяяяяяяяяяяяяяяяяяяяяяЂяяяяяяяяяяяяяяяяяяяяяяяяяяяяяяяяяяяяяяяяяяяяяяяяяяяяяяяяяяяяяяяяяяяяяяяяяяяяяяяяяяяяяяяяяяяяяяяяяяяяяяяяяяяяяяяяяяяяяяяяяяяяяяяяяяяяяяяяяяяяяяяяяяяяяяяяяяяяяяяяяяяяяяяяяяяяяяяяяяяяяяяяяяяяяяяяяяяяяяяяяяяяяяяяяяяяяяяяяяяяяяяяяяяяяяяяяяяяяяяяяяяяяяяяяяяяяяяяяяЂяяяяяяяяяяяяяяяяяяяяяяяяяяяяяяяяяяяяяяяяяяяяяяяяяяяяяяяяяяяяяяяяяЂяяяяяяяяяяяяяяяяяяяяяяяяяяяяяяяяяяяяяяяяяяяяяяяяяяяяяяяяяяяяяяяяяАяяяяяяяяяяяяяяяяяяяяяяяяяяяяяяяяяяяяяяяяяяяяяяяяяяяяяяяяяяяяяяяяяАяяяяяяяяяяяяяяяяяяяяяяяяяяяяяяяяяяяяяяяяяяяяяяяяяяяяяяяяяяяяяяяяяа?яяяяяяяяяяяяяяяяяяяяяяяяяяяяяяяяяяяяяяяяяяяяяяяяяяяяяяяяяяяяяяяяяаяяяяяяяяяяяяяяяяяяяяяяяяяяяяяяяяяяяяяяяяяяяяяяяяяяяяяяяяяяяяяяяяяяуяяяяяя"
  # "LOGO FASmedic en noir et blanc rotation180°"
  # "GW265,824,32,61,яяяяяяяяяяяяяяяяяяяяяяяяяяяяяяяЏяяяяяяяяяяяяяяяяяяяяяяяяяяяяяяюяяяяяяяяяяяяяяяяяяяяяяяяяяяяяяшяяяяяяяяяяяяяяяяяяяяяяяяяяяяяяАяяяяяяяяяяяяяяяяяяяяяяяяяяяяяяяяяяяяяяяяяяяяяяяяяяяяяяяяяяяяяяяяяяяяяяяяяяяяяяяяяяяяяяяяяюяяяяяяяяяяяяяяяяяяяяяяяяяяяяяюяяяяяяяяяяяяяяяяяяяяяяяяяяяяяюяяяяяяяяяяяяяяяяяяяяяяяяяяяяяьяяяяяяяяяяяяяяяяяяяяяяяяяяяяяьяяяяяяяяяяяяяяяяяяяяяяяяяяяяяшяЃяяяяьяяяяяяаяяяЂ?яяяяяяяшюП<ярьящяуя?Аяю8ш>П0x?БрьящяуьАяь0щяЏП#яЏь|ящяушАяшpуяЗП'яЏю<ящяурАяр`гягПяЏ?яящяуарАшяаазяуПяЗ?яњящяуашАьяЂАЗяуПяж?яњящяуашАьяАПяыПяжяЬящяуаяяАья~АяящПязяяМящяуаяяАшяЂяящП?язяяМящяуаяАаяЂяящП?ячяяМящяур?АяЂ?яящП?яцящяурАяА?яящП?яцящяушАяаяящП?яжяМящяуяАяряящПяжяЬящяуярАяяряяыПяжяњящягяяаАяяяшяПяуПяж?яњящягррАяяяяяяяяяяЗяуПяЗ?яясягррАшяяяяяяязягПяП?я>ясягрраряЂягязП'яЏџю>аяГраяЂ0ясяЏП#я‡ь~?А“шря0яшяП1ь?ГряЊ3ьшюpяь?П8аяЂsьью`яяЃяя?ѓяюяаяГяяАяяАяяьаяяяяя?яяяяяяяяяяяяяяяяяяьАяяяяя?яяяяяяяяяяяяяяяяяюьАяяяяя?яяяяяяяяяяяяяяяяяюшАяяяяя?яяяяяяяяяяяяяяяяяьшЂяяяяП?яяяяяяяяяяяяяяяяярЂяяяяП?яяяяяяяяяяяяяяяяяяр?яяяяП?яяяяяяяяяяяяяяяяяяр?яяяяП?яяяяяяяяяяяяяяяяяяаяяяяП?яяяяяяяяяяяяяяяяяяаяяяяяяяяяяяяяяяяяяяяяяяяАяяяяяяяяяяяяяяяяяяяяяяяяяяяАяяяяяяяяяяяяяяяяяяяяяяяяяяяЂяяяяяяяяяяяяяяяяяяяяяяяяяяяяяЂяяяяяяяяяяяяяяяяяяяяяяяяяяяяяЂ?яяяяяяяяяяяяяяяяяяяяяяяяяяяяяЂ?яяяяяяяяяяяяяяяяяяяяяяяяяяяяяЂ?яяяяяяяяяяяяяяяяяяяяяяяяяяяяяЂяяяяяяяяяяяяяяяяяяяяяяяяяяяяяАяяяяяяяяяяяяяяяяяяяяяяяяяяяяяаяяяяяяяяяяяяяяяяяяяяяяяяяяяяяяаяяяяяяяяяяяяяяяяяяяяяяяяяяяяяяряяяяяяяяяяяяяяяяяяяяяяяяяяяяяяр?яяяяяяяяяяяяяяяяяяяяяяяяяяяяяяшяяяяяяяяяяяяяяяяяяяяяяяяяяяяяящяяяяяя"
  # "Petite etiquette"
  # "ZB\nUS\nq600\nD7\nN\nR150,20\nI8,12,001\nA0,40,0,2,1,1,N,\"Carton : 1/1\"\nA0,85,0,2,1,1,N,\"Nb de valves : 25\"\nA0,130,0,2,1,1,N,\"Nø valves :\"\nA144,130,0,1,1,1,N,\"08120001, 08120002, 08120003, 08120004\"\nA144,146,0,1,1,1,N,\"08120005, 08120006, 08120007, 08120008\"\nA144,162,0,1,1,1,N,\"08120009, 08120010, 08120011, 08120012\"\nA144,178,0,1,1,1,N,\"08120013, 08120014, 08120015, 08120016\"\nA144,194,0,1,1,1,N,\"08120017, 08120018, 08120019, 08120020\"\nA144,210,0,1,1,1,N,\"08120021, 08120022, 08120023, 08120024\"\nA144,226,0,1,1,1,N,\"08120025\"\nB64,260,0,1,1,20,56,N,\"12-216C-04520 EQIFIL 104mA 36ohms\"\nA58,324,0,3,1,1,N,\"12-216C-04520 EQIFIL 104mA 36\"\nA466,321,0,4,1,1,N,\"Õ\""
  # "Test sens codes bar"
  # "ZB\nUS\nq592\nD7\nN\nR166,48\nI8,12,001\nB0,0,0,1,1,2,56,B,\"12-216C-04521 EQIFIL 417mA 14.4ohms\"\nB400,200,2,1,1,2,56,B,\"12-216C-04521 EQIFIL 417mA 14.4ohms\"\nB300,800,3,1,1,2,56,B,\"12-216C-04521 EQIFIL 417mA 14.4ohms\"\nB200,350,1,1,1,2,56,B,\"12-216C-04521 EQIFIL 417mA 14.4ohms\"\nP1"
  # "(2)"
  # "(8)"
  # "(17)"
  # "code bar fixe + indice  n° commande"
  # "1121057400 01054/08-01.01.01"
  # "code 39 client"
  # "B406,128,2,3,1,2,56,N,\"MK3845ZZ45988 03 08120812 25\""
  # "code 128 client"
  # "B406,128,2,1,1,20,56,N,\"MK3845ZZ45988 03 08120812 25\""
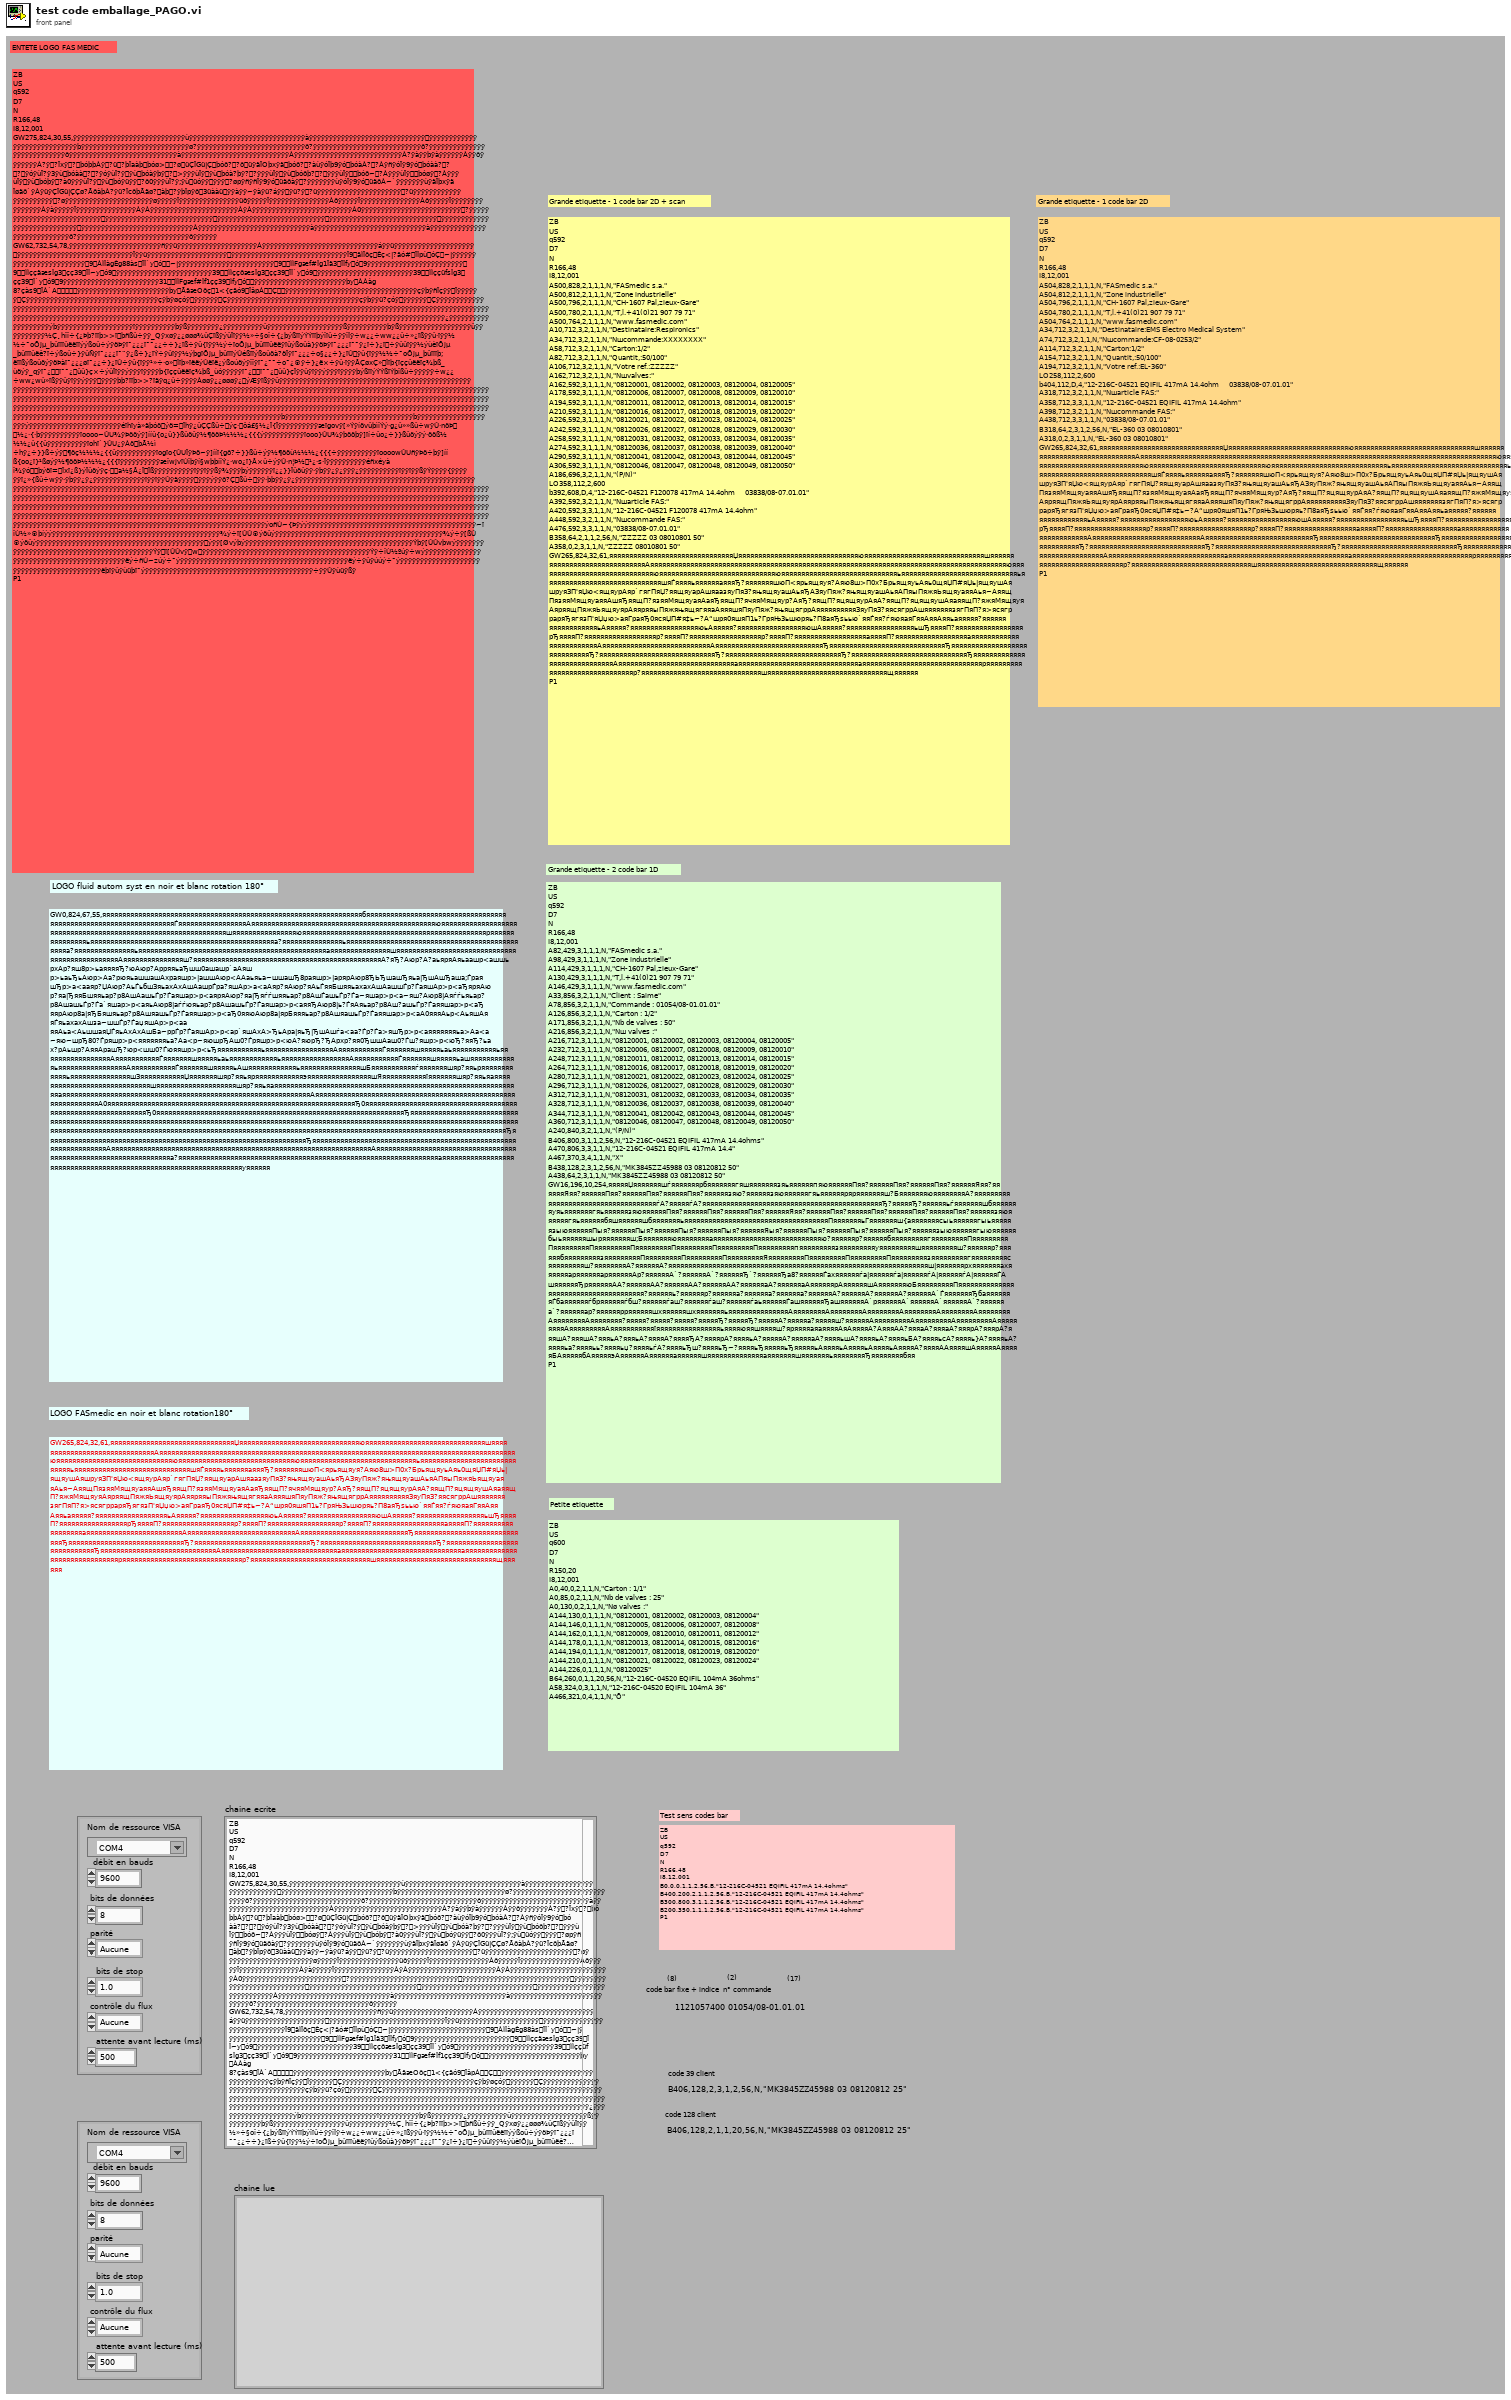
[diagram p1: front panel]
types:
  T1 = cluster{"VISA resource name":refnum<visa-resource-name>, "baud rate":u32, "data bits":u16, "parity":u16, "stop bits":u16, "flow control":u16, "delay before read (ms)":u32}
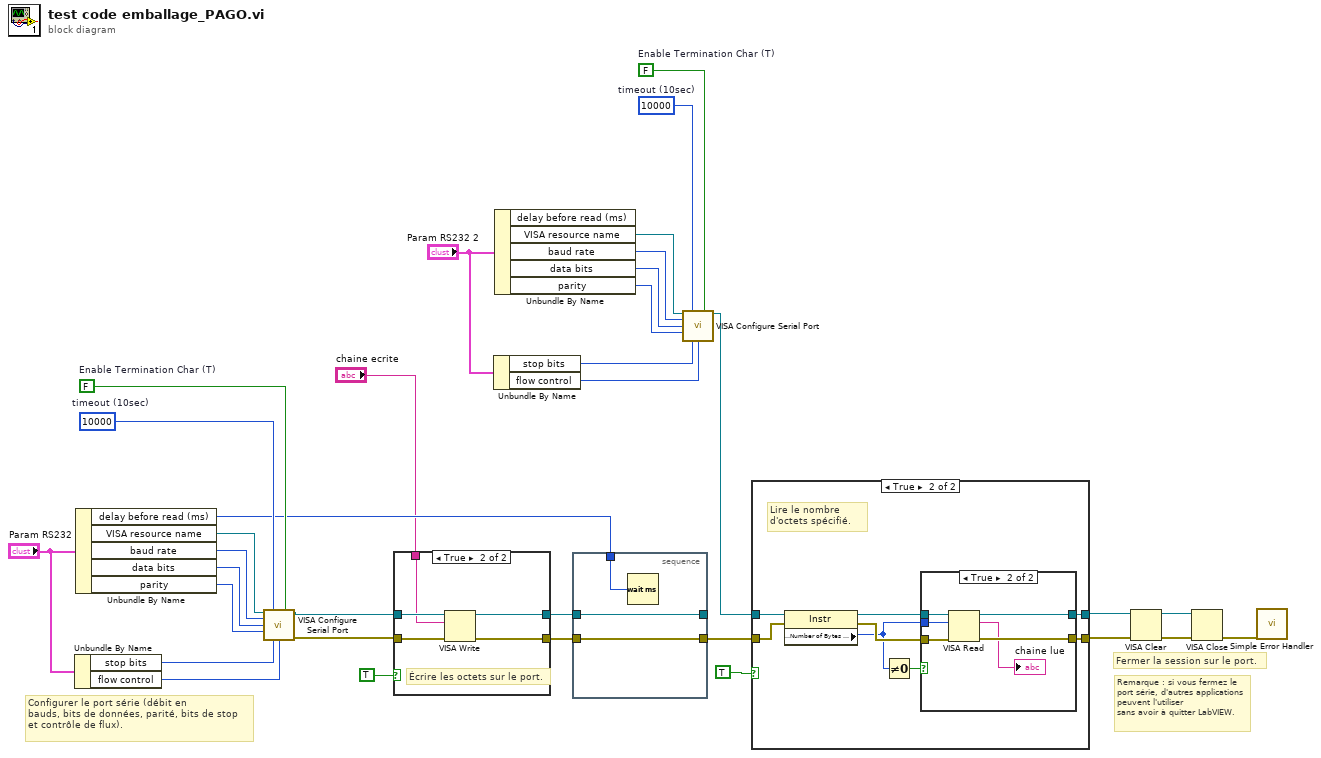
[diagram p0: block diagram]
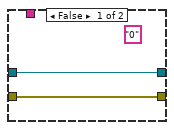
[diagram p2: hidden frame]
diagram:
  w6 = FALSE  # Enable Termination Char (T)
  w7 = u32 10000  # timeout (10sec)
  w32 = FALSE  # Enable Termination Char (T)
  w33 = u32 10000  # timeout (10sec)
  # "Remarque : si vous fermez le port série, d'autres applications peuvent l'utiliser\nsans avoir à quitter LabVIEW."
  # "Fermer la session sur le port."
  # "Configurer le port série (débit en\nbauds, bits de données, parité, bits de stop\net contrôle de flux)."
  n1 = Unbundle By Name("Param RS232") -> ("stop bits"=w26:u16, "flow control"=w25:u16)
  n2 = Unbundle By Name("Param RS232") -> ("delay before read (ms)"=w18:u32, "VISA resource name"=w31:refnum<visa-resource-name>, "baud rate"=w30:u32, "data bits"=w29:u16, "parity"=w28:u16)
  n3 = call-poly "VISA Configure Serial Port"("VISA resource name"=w31, "timeout (10sec)"=w33, "Enable Termination\nChar (T)"=w32, "baud rate (9600)"=w30, "data bits (8)"=w29, "parity (0:none)"=w28, "stop bits (10: 1 bit)"=w26, "flow control (0:none)"=w25) -> ("VISA resource name out"=w17:refnum<visa-resource-name>, "error out"=w16:errorcluster)  [unwired: 6 in]
  n4 = case shown="True" TRUE {
    tunnel: [w35 w40] -> w23
    tunnel: w17 -> [w34 w39]
    tunnel: w16 -> [w35 w38]
    tunnel: [w34 w37] -> w21
    tunnel: "chaine ecrite" -> [_ w36]
    frame False {
      (unwired) "0" ("string to write")
    }
    frame True {
      # "Écrire les octets sur le port."
      n5 = VISA Write(VISA resource name=w39, write buffer=w36, error in (no error)=w38) -> (VISA resource name out=w37:refnum<visa-resource-name>, error out=w40:errorcluster)  [unwired: 1 out]
    }
  }
  n6 = Unbundle By Name("Param RS232 2") -> ("stop bits"=w9:u16, "flow control"=w8:u16)
  n7 = Unbundle By Name("Param RS232 2") -> ("VISA resource name"=w14:refnum<visa-resource-name>, "baud rate"=w13:u32, "data bits"=w12:u16, "parity"=w11:u16)  [unwired: 1 out]
  n8 = stacked-sequence {
    tunnel: w23 -> [w43]
    tunnel: [w43] -> w22
    tunnel: w21 -> [w42]
    tunnel: [w42] -> _
    tunnel: w18 -> [w41]
    frame #0 {
      n9 = Wait (ms)(milliseconds to wait=w41) -> ()  [unwired: 1 out]
    }
  }
  n10 = call-poly "VISA Configure Serial Port"("VISA resource name"=w14, "timeout (10sec)"=w7, "Enable Termination\nChar (T)"=w6, "baud rate (9600)"=w13, "data bits (8)"=w12, "parity (0:none)"=w11, "stop bits (10: 1 bit)"=w9, "flow control (0:none)"=w8) -> ("VISA resource name out"=w5:refnum<visa-resource-name>)  [unwired: 6 in, 1 out]
  n11 = case shown="True" TRUE ("Booléen") {
    tunnel: w22 -> [w45 w49]
    tunnel: [w45 w53] -> w3
    tunnel: [w44 w52] -> w4
    tunnel: w5 -> [w44 w51]
    frame False {
    }
    frame True {
      # "Lire le nombre d'octets spécifié."
      n12 = property class="Instr"(reference=w51, error in=w49) -> (reference out=w50:refnum<visa-resource-name>, error out=w48:errorcluster, "Serial Settings:Number of Bytes at Serial Port"=w46:u32)
      n13 = Not Equal To 0?(x=w46) -> (x != 0?=w47:bool)
      n14 = case shown="True" w47 {
        tunnel: [w55 w61] -> w53
        tunnel: [w54 w60] -> w52
        tunnel: w50 -> [w54 w59]
        tunnel: w48 -> [w55 w58]
        tunnel: w46 -> [_ w56]
        frame False {
        }
        frame True {
          n15 = VISA Read(VISA resource name=w59, byte count=w56, error in (no error)=w58) -> (VISA resource name out=w60:refnum<visa-resource-name>, read buffer=→"chaine lue":string, error out=w61:errorcluster)  [unwired: 1 out]
        }
      }
    }
  }
  n16 = VISA Clear(VISA resource name=w4, error in (no error)=w3) -> (VISA resource name out=w1:refnum<visa-resource-name>, error out=w2:errorcluster)
  n17 = VISA Close(VISA resource name=w1, error in (no error)=w2) -> (error out=w24:errorcluster)
  n18 = call <vilib>:"Simple Error Handler.vi"("error in (no error)"=w24) -> ()  [unwired: 4 in, 5 out]
